vi "HandleExit.vi"(8 "error in (no error)":errorcluster, 9 "VI Refnum":refnum<vi>, 10 "StopArgument":variant, 11 "ModuleAdmin":refnum<class "ModuleAdmin.lvclass">) -> (0 "error out":errorcluster, 1 "Exit via Stop Module Req?":bool, 2 "WaitForStop?":bool)   [LabVIEW 2018, in "AcPwrPlugins.lvlib"]
doc: "This VI hides Main.vi if it was externally launched and extracts the conditions of the closing."
uses:
  AcPwrPlugins.lvlib
  <userlib>/NIST/ModuleAdminLib/ModuleAdmin/ModuleAdmin.lvclass
  C:/Program Files (x86)/National Instruments/LabVIEW 2018/user.lib/NIST/ModuleAdminLib/ModuleAdminBase/ModuleAdminBase.lvclass
  AcPwrShared/clStopArgument.ctl
  AcPwrShared/AcPwrShared.lvlib
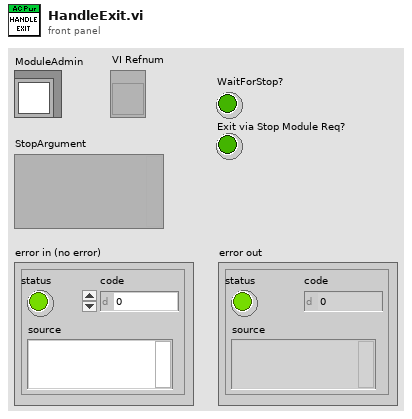
[diagram p1: front panel]
types:
  T1 = typedef "AcPwrShared.lvlib/clStopArgument.ctl" = cluster{"Exit via Stop Module Req?":bool, "Wait for Module to stop?":bool, "ModuleAdmin":refnum<class "ModuleAdmin.lvclass">}
  T2 = enum32{"Invalid", "Standard", "Closed", "Hidden", "Minimized", "Maximized"}
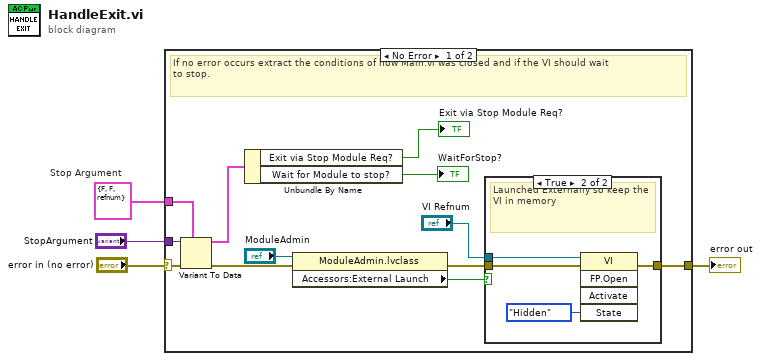
[diagram p0: block diagram]
diagram:
  w3 = T1 {"Exit via Stop Module Req?"=FALSE, "Wait for Module to stop?"=FALSE, "ModuleAdmin"=refnum}  # Stop Argument
  n1 = case shown="No Error" "error in (no error)" {
    selector: "error in (no error)" -> [w7 w22]
    tunnel: [w15 w22] -> w4
    tunnel: w3 -> [w14 _]
    tunnel: "StopArgument" -> [w12 _]
    frame No Error {
      # "If no error occurs extract the conditions of how Main.vi was closed and if the VI should wait\nto stop."
      n2 = Variant To Data(error in=w7, type=w14, Variant=w12) -> (data=w13:T1, error out=w6:errorcluster)
      n3 = Unbundle By Name(w13) -> ("Exit via Stop Module Req?"=→"Exit via Stop Module Req?":bool, "Wait for Module to stop?"=→"WaitForStop?":bool)
      n4 = property class="ModuleAdmin.lvclass"(reference="ModuleAdmin", error in=w6) -> (error out=w5:errorcluster, "Accessors:External Launch"=w11:bool)  [unwired: 1 out]
      n5 = case shown="True" w11 {
        tunnel: "VI Refnum" -> [_ w21]
        tunnel: [w17 w19] -> w15
        tunnel: w5 -> [w17 w18]
        frame False {
        }
        frame True {
          # "Launched Externally so keep the VI in memory"
          n6 = invoke class="VI" method="FP.Open"(reference=w21, error in=w18, "State"=T2."Hidden") -> (error out=w19:errorcluster)  [unwired: 2 in, 4 out]
        }
      }
    }
    frame Error {
    }
  }
  "error out" <- w4
